vi "Coumtdown Timer.vi"() -> ()   [LabVIEW 2017]
panel:
  out "Minutes":i32
  out "Hours":i32
  out "Seconds":i32
  in  "Seconds to Wait":i32=1000
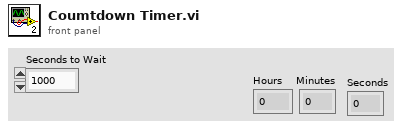
[diagram p1: front panel]
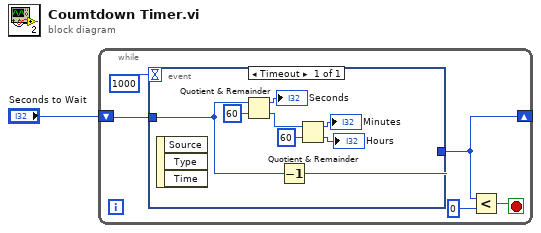
[diagram p0: block diagram]
diagram:
  n1 = while {
    shift-right: [w3] -> _
    shift-left: "Seconds to Wait" -> [w5]
    stop <- w4 stop-if-true
    n2 = event shown="[0] Timeout" {
      selector: _ -> [_]
      dyn-events: _ -> [_]
      timeout: 1000 -> [_]
      tunnel: w5 -> [w12]
      tunnel: [w14] -> w3
      event Timeout {
        n3 = event-data() -> ()  [unwired: 1 in, 3 out]
        n4 = Quotient & Remainder(x=w12, y=60) -> (x-y*floor(x/y)=→"Seconds":i32, floor(x/y)=w8:i32)
        n5 = Decrement(x=w12) -> (x-1=w14:i32)
        n6 = Quotient & Remainder(x=w8, y=60) -> (x-y*floor(x/y)=→"Minutes":i32, floor(x/y)=→"Hours":i32)
      }
    }
    n7 = Less?(x=w3, y=0) -> (x < y?=w4:bool)
  }
